vi "USBcam_liveview.vi"() -> ()   [LabVIEW 2020]
uses:
  <vilib>/userDefined/High Color/IMAQdx.ctl
  <vilib>/vision/driver/IMAQdx.llb/IMAQdx Buffer Number Mode.ctl
  <vilib>/vision/driver/NI_Vision_Acquisition_Software.lvlib
panel:
  in  "Buffer Number Mode (Next)":T1
  in  "error constant":errorcluster
  in  "stop":bool
  in  "USB camera":T2
  out "Image":T3(plugin-control)
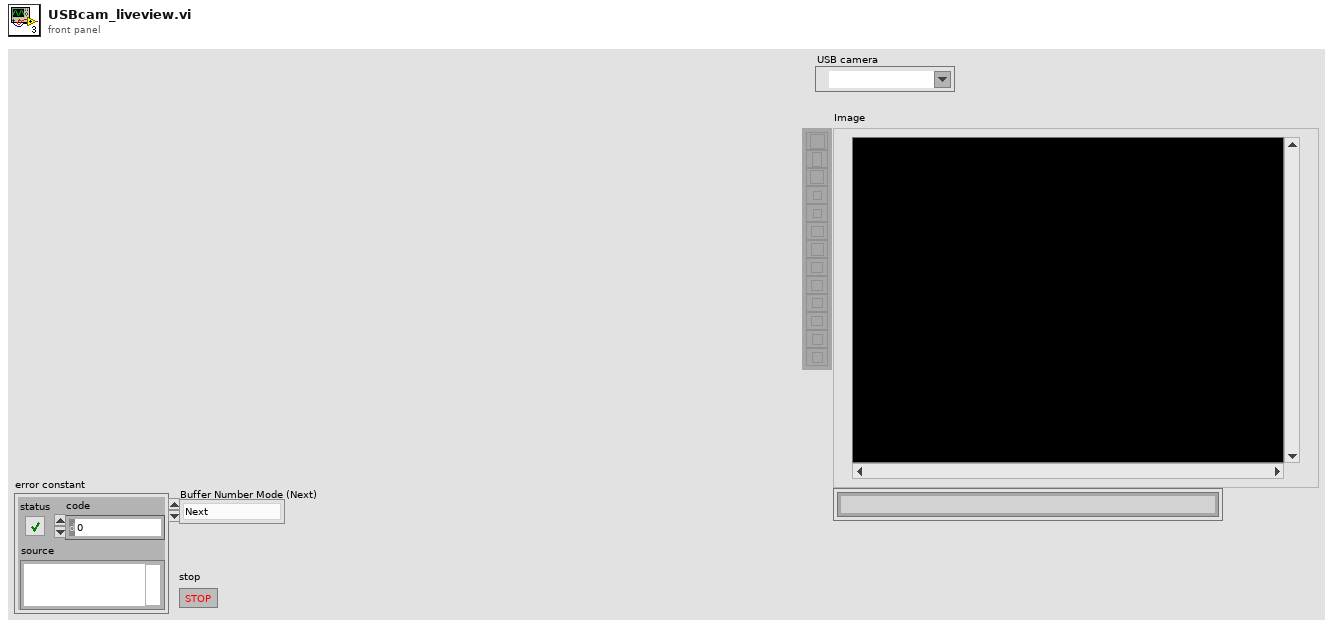
[diagram p1: front panel]
types:
  T1 = typedef "NI_Vision_Acquisition_Software.lvlib/IMAQdx Buffer Number Mode.ctl" = enum32{"Next", "Last", "Buffer Number", "Every", "Last New"}
  T2 = typedef "IMAQdx.ctl" = refnum<k21>
  T3 = typedef "IMAQ Image.ctl" = refnum<image>
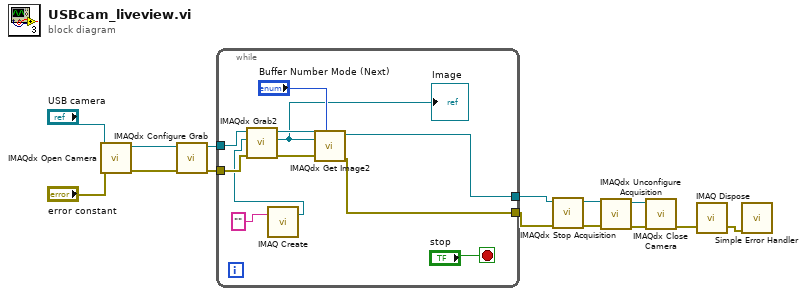
[diagram p0: block diagram]
diagram:
  n1 = call <vilib>:"IMAQdx Open Camera.vi"("error in"="error constant", "Session In"="USB camera") -> ("error out"=w12:errorcluster, "Session Out"=w13:T2)  [unwired: 8 in]
  n2 = call <vilib>:"IMAQdx Configure Grab.vi"("error in"=w12, "Session In"=w13) -> ("error out"=w2:errorcluster, "Session Out"=w4:T2)  [unwired: 8 in]
  n3 = while {
    tunnel: [w18] -> w5
    tunnel: w4 -> [w21]
    tunnel: [w22] -> w3
    tunnel: w2 -> [w24]
    stop <- "stop" stop-if-true
    n4 = call "IMAQ Create"("Image Name"="") -> ("New Image"=w15:T3)  [unwired: 4 in, 1 out]
    n5 = call <vilib>:"IMAQdx Grab2.vi"("error in"=w24, "Image In"=w15, "Session In"=w21) -> ("error out"=w19:errorcluster, "Image Out"=w20:T3, "Session Out"=w25:T2)  [unwired: 5 in, 1 out]
    "Image" <- w20
    n6 = call <vilib>:"IMAQdx Get Image2.vi"("Buffer Number Mode (Next)"="Buffer Number Mode (Next)", "error in"=w19, "Image In"=w20, "Session In"=w25) -> ("error out"=w18:errorcluster, "Session Out"=w22:T2)  [unwired: 4 in, 2 out]
  }
  n7 = call <vilib>:"IMAQdx Stop Acquisition.vi"("error in"=w5, "Session In"=w3) -> ("error out"=w11:errorcluster, "Session Out"=w10:T2)  [unwired: 8 in]
  n8 = call <vilib>:"IMAQdx Unconfigure Acquisition.vi"("error in"=w11, "Session In"=w10) -> ("error out"=w9:errorcluster, "Session Out"=w8:T2)  [unwired: 8 in]
  n9 = call <vilib>:"IMAQdx Close Camera.vi"("error in"=w9, "Session In"=w8) -> ("error out"=w7:errorcluster)  [unwired: 9 in]
  n10 = call "IMAQ Dispose"("error in (no error)"=w7) -> ("error out"=w6:errorcluster)  [unwired: 5 in]
  n11 = call <vilib>:"Simple Error Handler.vi"("error in (no error)"=w6) -> ()  [unwired: 4 in, 5 out]
